vi "Get Earths Eccentricity.vi"(11 "Julian Century":dbl) -> (3 "Eccentricity":dbl)   [LabVIEW 2014, in "Solar Calculations.lvlib"]
uses:
  Solar Calculations.lvlib
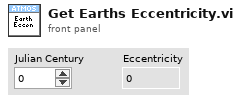
[diagram p1: front panel]
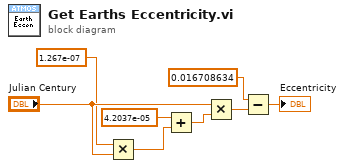
[diagram p0: block diagram]
diagram:
  n1 = Multiply(x=1.267e-07, y="Julian Century") -> (x*y=w2:dbl)
  n2 = Add(x=4.2037e-05, y=w2) -> (x+y=w4:dbl)
  n3 = Multiply(x="Julian Century", y=w4) -> (x*y=w6:dbl)
  n4 = Subtract(x=0.016708634, y=w6) -> (x-y=→"Eccentricity":dbl)
